vi "John digital out control.vi"() -> ()   [LabVIEW 2017]
uses:
  <vilib>/DAQmx/write.llb/DAQmx Write (Digital Bool 1Line 1Point).vi
  <vilib>/DAQmx/create/channels.llb/DAQmx Create Channel (DO-Digital Output).vi
  <vilib>/DAQmx/miscellaneous.llb/DAQmx Fill In Error Info.vi
panel:
  in  "Clear all outputs":bool
  out "Current channel 2":bool
  out "Current channel 1":bool
  out "Current channel 0":bool
  in  "Set outputs":bool
  in  "Channel 2":bool
  in  "Channel 1":bool
  in  "Channel 0":bool
  in  "stop":bool
  # "on"
  # "off"
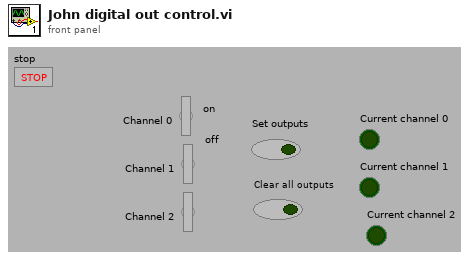
[diagram p1: front panel]
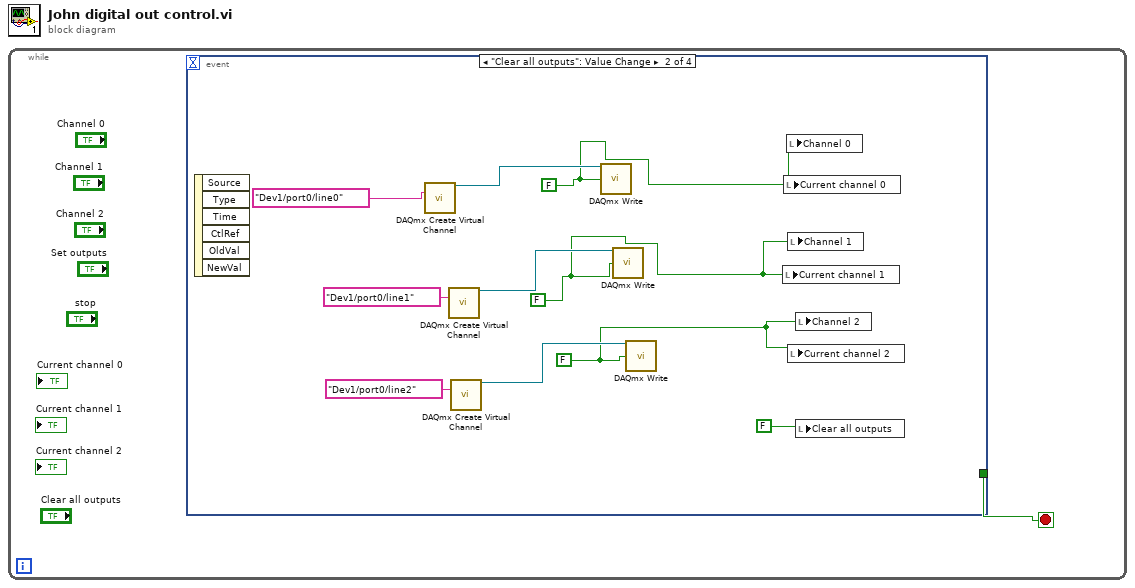
[diagram p0: block diagram]
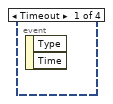
[diagram p2: hidden frame]
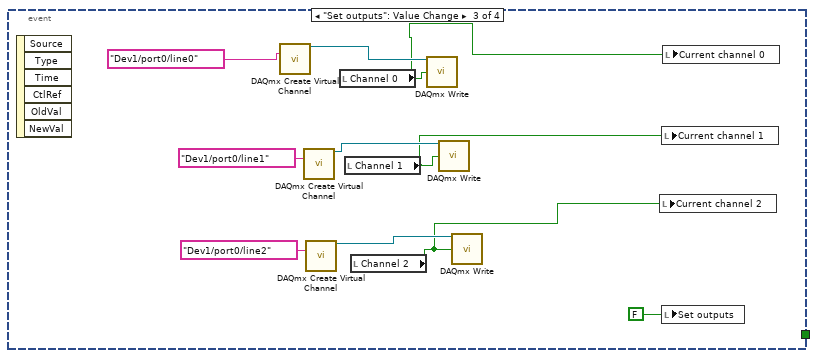
[diagram p3: hidden frame]
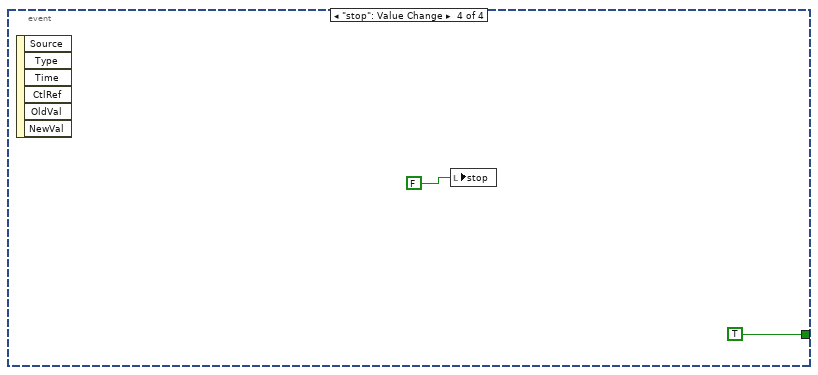
[diagram p4: hidden frame]
diagram:
  n1 = while {
    stop <- w1 stop-if-true
    n2 = event shown="[1] \"Clear all outputs\": Value Change" {
      selector: _ -> [_ _ _ _]
      dyn-events: _ -> [_ _ _ _]
      timeout: _ -> [_ _ _ _]
      tunnel: [_ _ _ TRUE] -> w1
      event Timeout {
        n3 = event-data() -> ()  [unwired: 3 out]
      }
      event "Clear all outputs": Value Change {
        w4 = FALSE
        w3 = FALSE
        w2 = FALSE
        n4 = event-data() -> ()  [unwired: 7 out]
        n5 = call-poly <vilib>:"DAQmx Create Virtual Channel.vi"("lines"=tag "Dev1/port0/line0") -> ("task out"=w8:refnum<k21>)  [unwired: 5 in, 9 out]
        n6 = call-poly <vilib>:"DAQmx Create Virtual Channel.vi"("lines"=tag "Dev1/port0/line1") -> ("task out"=w7:refnum<k21>)  [unwired: 5 in, 9 out]
        n7 = call-poly <vilib>:"DAQmx Create Virtual Channel.vi"("lines"=tag "Dev1/port0/line2") -> ("task out"=w6:refnum<k21>)  [unwired: 5 in, 9 out]
        n8 = call-poly <vilib>:"DAQmx Write.vi"("task/channels in"=w8, "data"=w2) -> ()  [unwired: 2 in, 12 out]
        n9 = call-poly <vilib>:"DAQmx Write.vi"("task/channels in"=w7, "data"=w3) -> ()  [unwired: 2 in, 12 out]
        n10 = call-poly <vilib>:"DAQmx Write.vi"("task/channels in"=w6, "data"=w4) -> ()  [unwired: 2 in, 12 out]
        n11 = local write "Current channel 1"(w3) -> ()
        n12 = local write "Current channel 0"(w2) -> ()
        n13 = local write "Channel 0"(w2) -> ()
        n14 = local write "Channel 1"(w3) -> ()
        n15 = local write "Current channel 2"(w4) -> ()
        n16 = local write "Channel 2"(w4) -> ()
        n17 = local write "Clear all outputs"(FALSE) -> ()
      }
      event "Set outputs": Value Change {
        n18 = event-data() -> ()  [unwired: 7 out]
        n19 = call-poly <vilib>:"DAQmx Create Virtual Channel.vi"("lines"=tag "Dev1/port0/line0") -> ("task out"=w21:refnum<k21>)  [unwired: 5 in, 9 out]
        n20 = call-poly <vilib>:"DAQmx Create Virtual Channel.vi"("lines"=tag "Dev1/port0/line1") -> ("task out"=w18:refnum<k21>)  [unwired: 5 in, 9 out]
        n21 = call-poly <vilib>:"DAQmx Create Virtual Channel.vi"("lines"=tag "Dev1/port0/line2") -> ("task out"=w17:refnum<k21>)  [unwired: 5 in, 9 out]
        n22 = local read "Channel 0"() -> (w14:bool)
        n23 = local read "Channel 1"() -> (w13:bool)
        n24 = local read "Channel 2"() -> (w12:bool)
        n25 = call-poly <vilib>:"DAQmx Write.vi"("task/channels in"=w21, "data"=w14) -> ()  [unwired: 2 in, 12 out]
        n26 = call-poly <vilib>:"DAQmx Write.vi"("task/channels in"=w18, "data"=w13) -> ()  [unwired: 2 in, 12 out]
        n27 = call-poly <vilib>:"DAQmx Write.vi"("task/channels in"=w17, "data"=w12) -> ()  [unwired: 2 in, 12 out]
        n28 = local write "Current channel 2"(w12) -> ()
        n29 = local write "Current channel 1"(w13) -> ()
        n30 = local write "Set outputs"(FALSE) -> ()
        n31 = local write "Current channel 0"(w14) -> ()
      }
      event "stop": Value Change {
        n32 = event-data() -> ()  [unwired: 7 out]
        n33 = local write "stop"(FALSE) -> ()
      }
    }
  }
